vi "Strain Conversion.vi"(0 "Current Wavelength (0 nm)":dbl format="%#_10g", 1 "Nominal Wavelength (0 nm)":dbl format="%#_10g", 5 "Temperature Change (°C)":dbl, 7 "CTE of Test Specimen (0)":dbl, 9 "Gage Factor (0.89)":dbl=0.89, 11 "Gage Constant 1 (6.156)":dbl=6.156, 12 "Gage Constant 2 (0.7)":dbl=0.7) -> (6 "Strain (µm/m)":dbl)   [LabVIEW 2015, in "Micron Optics sm130.lvlib"]
doc: "Converts the wavelength shift to strain measurement.\n\n<b>Note:</b>\n1.) This conversion VI is compatible with Micron Optics sensor model os3110, os3120, os3200, os3600.\n2.) Refer to the Sensor Information Sheet provided with each sensor for the constants."
uses:
  Micron Optics sm130.lvlib
panel:
  # "This conversion VI is compatible with Micron Optics sensor model os3110, os3120, os3200 and os3600."
  # "Constants"
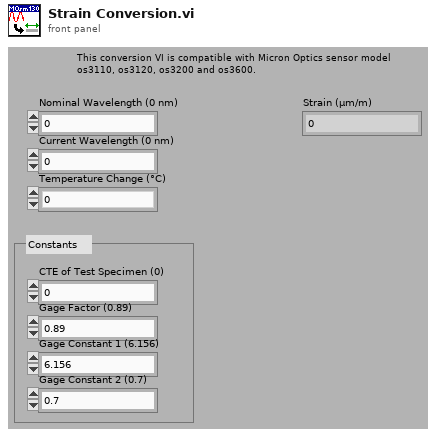
[diagram p1: front panel]
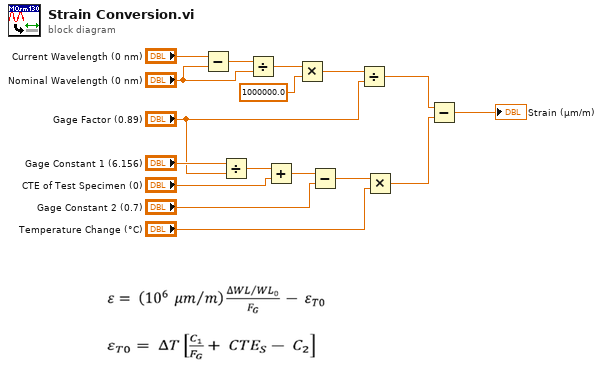
[diagram p0: block diagram]
diagram:
  n1 = Subtract(x="Current Wavelength (0 nm)", y="Nominal Wavelength (0 nm)") -> (x-y=w16:dbl)
  n2 = Divide(x="Gage Constant 1 (6.156)", y="Gage Factor (0.89)") -> (x/y=w9:dbl)
  n3 = Divide(x=w16, y="Nominal Wavelength (0 nm)") -> (x/y=w14:dbl)
  n4 = Add(x=w9, y="CTE of Test Specimen (0)") -> (x+y=w7:dbl)
  n5 = Multiply(x=w14, y=1000000.0) -> (x*y=w12:dbl)
  n6 = Subtract(x=w7, y="Gage Constant 2 (0.7)") -> (x-y=w5:dbl)
  n7 = Divide(x=w12, y="Gage Factor (0.89)") -> (x/y=w3:dbl)
  n8 = Multiply(x=w5, y="Temperature Change (°C)") -> (x*y=w2:dbl)
  n9 = Subtract(x=w3, y=w2) -> (x-y=→"Strain (µm/m)":dbl)
